vi "trafic light.vi"() -> ()   [LabVIEW 2018]
panel:
  in  "stop":bool
  out "red":bool
  out "yellow":bool
  out "green":bool
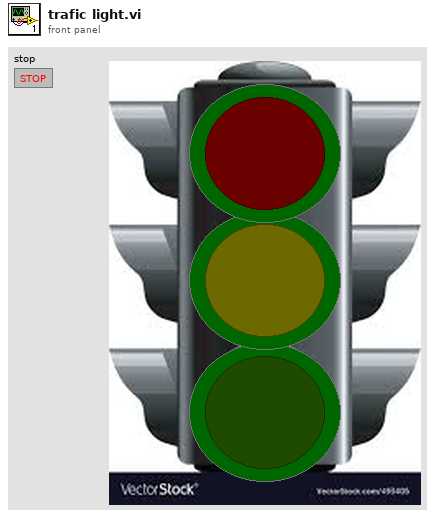
[diagram p1: front panel]
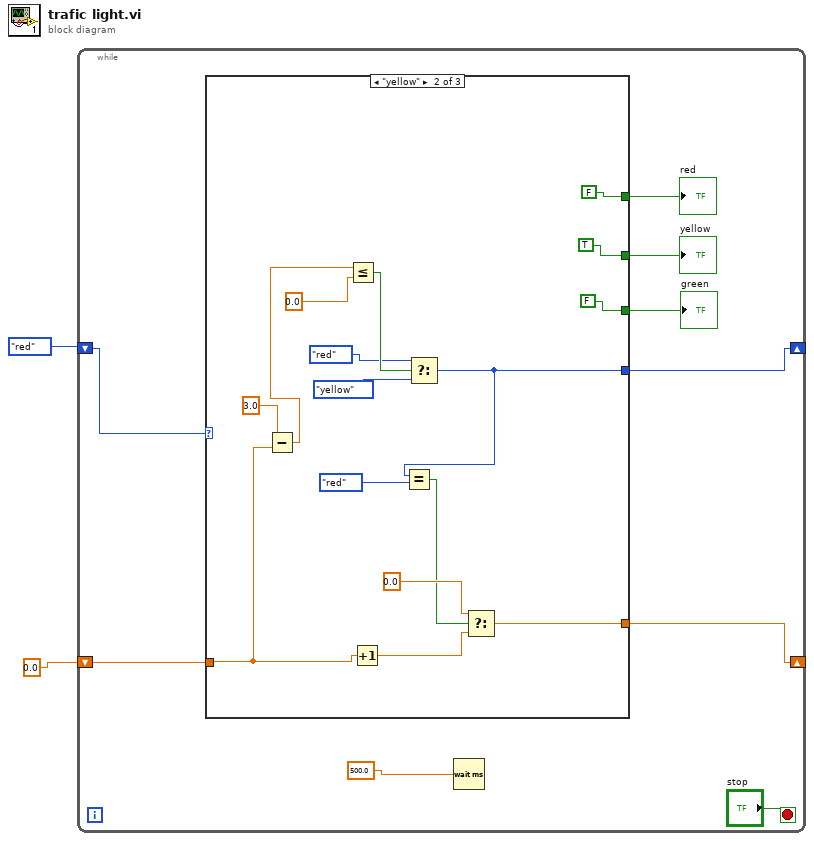
[diagram p0: block diagram]
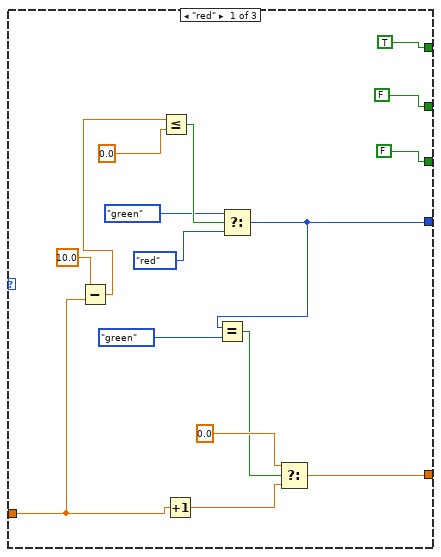
[diagram p2: hidden frame]
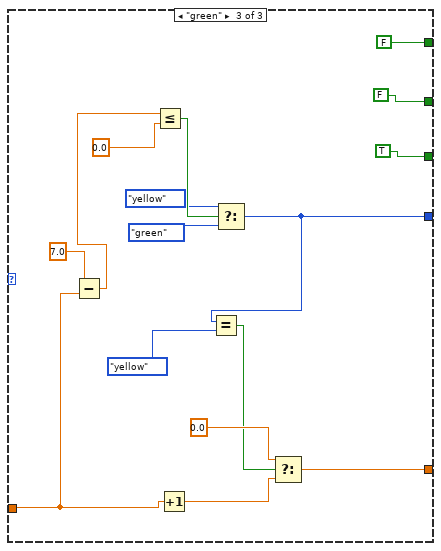
[diagram p3: hidden frame]
diagram:
  n1 = while {
    shift-right: [w8] -> _
    shift-left: enum16{"green", "yellow", "red"}."red" -> [w11]
    shift-right: [w9] -> _
    shift-left: 0.0 -> [w10]
    stop <- "stop" stop-if-true
    n2 = case shown="\"yellow\"" w11 {
      tunnel: w10 -> [w23 w36 w50]
      tunnel: [w26 w35 w51] -> w9
      tunnel: [w18 w34 w52] -> w8
      tunnel: [TRUE FALSE FALSE] -> w7
      tunnel: [FALSE TRUE FALSE] -> w6
      tunnel: [FALSE FALSE TRUE] -> w5
      frame "red" {
        n3 = Subtract(x=10.0, y=w23) -> (x-y=w21:dbl)
        n4 = Less Or Equal?(x=w21, y=0.0) -> (x <= y?=w19:bool)
        n5 = Increment(x=w23) -> (x+1=w27:dbl)
        n6 = Select(t=enum16{"green", "yellow", "red"}."green", s=w19, f=enum16{"green", "yellow", "red"}."red") -> (s? t:f=w18:enum16{"green", "yellow", "red"})
        n7 = Equal?(x=w18, y=enum16{"green", "yellow", "red"}."green") -> (x = y?=w24:bool)
        n8 = Select(t=0.0, s=w24, f=w27) -> (s? t:f=w26:dbl)
      }
      frame "yellow" {
        n9 = Subtract(x=3.0, y=w36) -> (x-y=w39:dbl)
        n10 = Less Or Equal?(x=w39, y=0.0) -> (x <= y?=w37:bool)
        n11 = Increment(x=w36) -> (x+1=w43:dbl)
        n12 = Select(t=enum16{"green", "yellow", "red"}."red", s=w37, f=enum16{"green", "yellow", "red"}."yellow") -> (s? t:f=w34:enum16{"green", "yellow", "red"})
        n13 = Equal?(x=w34, y=enum16{"green", "yellow", "red"}."red") -> (x = y?=w41:bool)
        n14 = Select(t=0.0, s=w41, f=w43) -> (s? t:f=w35:dbl)
      }
      frame "green" {
        n15 = Subtract(x=7.0, y=w50) -> (x-y=w55:dbl)
        n16 = Less Or Equal?(x=w55, y=0.0) -> (x <= y?=w53:bool)
        n17 = Increment(x=w50) -> (x+1=w59:dbl)
        n18 = Select(t=enum16{"green", "yellow", "red"}."yellow", s=w53, f=enum16{"green", "yellow", "red"}."green") -> (s? t:f=w52:enum16{"green", "yellow", "red"})
        n19 = Equal?(x=w52, y=enum16{"green", "yellow", "red"}."yellow") -> (x = y?=w57:bool)
        n20 = Select(t=0.0, s=w57, f=w59) -> (s? t:f=w51:dbl)
      }
    }
    "green" <- w5
    "yellow" <- w6
    "red" <- w7
    n21 = Wait (ms)(milliseconds to wait=500.0) -> ()  [unwired: 1 out]
  }
